vi "GUI_Single Button Pump.vi"() -> ()   [LabVIEW 2011] (continued)
        n648 = call "Generate User Event.vi"("Add(t)/Remove(f) Event"=w1664, "error in (no error)"=w1676, "User Event in"=w1677, "Status Array In"=w1679, "Error Codes"=w1678) -> ("error out"=w1675:errorcluster)  [unwired: 5 in, 1 out]
        n649 = case shown="\"HPBD\"" w1673 {
          tunnel: [w1683 "M123 Roughing Valve is NOT open.\nPlease perform corrective action\n and click on continue.\nClick Exit to abort GPM" ("message") "HPBD Roughing Valve is NOT open.\nPlease perform corrective action\n and click on continue.\nClick Exit to abort GPM" ("message") "OAP Roughing Valve is NOT open.\nPlease perform corrective action\n and click on continue.\nClick Exit to abort GPM" ("message") w1690 "BTL Roughing Valve is NOT open.\nPlease perform corrective action\n and click on continue.\nClick Exit to abort GPM" ("message") "TARGET Roughing Valve is NOT open.\nPlease perform corrective action\n and click on continue.\nClick Exit to abort GPM" ("message") "BTL2 Roughing Valve is NOT open.\nPlease perform corrective action\n and click on continue.\nClick Exit to abort GPM" ("message") "HPD Roughing Valve is NOT open.\nPlease perform corrective action\n and click on continue.\nClick Exit to abort GPM" ("message")] -> w1668
          tunnel: [w1683 "Main: Check Roughing Valve Status>>M123" "Main: Check Roughing Valve Status>>HPBD" "Main: Check Roughing Valve Status>>OAP" w1690 "Main: Check Roughing Valve Status>>BTL" "Main: Check Roughing Valve Status>>TARGET" "Main: Check Roughing Valve Status>>BTL2" "Main: Check Roughing Valve Status>>HPD"] -> w1662
          frame "False", Default {
            w1683 = ""
          }
          frame "M123" {
          }
          frame "HPBD" {
          }
          frame "OAP" {
          }
          frame "COMP" {
            w1690 = ""
          }
          frame "BTL" {
          }
          frame "TARGET" {
          }
          frame "BTL2" {
          }
          frame "HPD" {
          }
        }
        n650 = call "MID-VAC Timer.vi"("Action"=timerAction_typdef."Timer Running") -> ("TO"=w1671:bool)  [unwired: 10 in]
        n651 = And(x=w1664, y=w1671) -> (x .and. y?=w1670:bool)
        n652 = call "Generate TO event.vi"("Boolean"=w1670, "message"=w1668, "User Event in"=w1669) -> ()  [unwired: 9 in]
        n653 = Unbundle By Name(w1667) -> ("VI Refnum"=w1666:refnum<vi>)
        n654 = control-ref of="User Input Panel"() -> (w1665:refnum<vi>)
        n655 = call "Gen Next State based on user input.vi"("Next State IN"="", "Generate Event?"=w1664, "Idle State"=w1662, "Continue To Wait State"=w1662, "VI Refnum"=w1666, "SubPanel in"=w1665) -> ("Next State Out"=w1661:string)  [unwired: 5 in]
        n656 = call <vilib>:"Add State(s) to Queue__jki_lib_state_machine.vi"("State(s) in Front (\"\")"=w1661, "State(s) in (\"\")"=w1682) -> ("States Out"=w1681:string)  [unwired: 13 in]
      }
      frame "---------- Main: Roughing Pumps----------" {
      }
      frame "Main: Start Roughing Pumps" {
        # "Open Roughing Pumps on both systems"
        n657 = Unbundle By Name(w1708) -> ("Debug Mode?"=w1707:bool)
        n658 = case shown="False" w1707 {
          tunnel: w1715 -> [w1722 w1728]
          tunnel: [w1719 w1728] -> w1714
          tunnel: w1708 -> [w1718 _]
          frame False {
            w1727 = T33[] [enum."LB Start Roughing Pump ", enum."EC Start Roughing Pump"] items=["No Action", "Set GPM Mode LB", "EXIT GPM Mode LB", "Set GPM Mode EC", "EXIT GPM Mode EC", "Set GVM mode LB", "Set GVM Mode EC", "Open LB Backing Valve", "Open EC Backing Valve", "Open EC Roughing Valve", "Open LB Roughing Valve", "Open M123 Roughing Valve", "Close M123 Roughing Valve", "Open Compressor Roughing Valve", "Close Compressor Roughing Valve", "Open BeamDump Roughing Valve", "Close BeamDump Roughing Valve", "Open OAP Roughing Valve", "Close OAP Roughing Valve", "Open BTL Roughing Valve", "Close BTL Roughing Valve", "Open Target Roughing Valve", "Close Target Roughing Valve", "Open BTL2 Roughing Valve", "Close BTL2 Roughing Valve", "Open HPD Roughing Valve", "Close HPD Roughing Valve", "LB Start Roughing Pump ", "EC Start Roughing Pump", "Open COMP Turbo Backing Valve", "Open M123 Turbo Backing Valve", "Open OAP Turbo Backing Valve", "Open HPBD Turbo Backing Valve", "Open BLT Turbo Backing Valve", "Open TARGET1 Turbo Backing Valve", "Open TARGET2 Turbo Backing Valve", "Open BLT2 Turbo Backing Valve", "Open HPD Turbo Backing Valve", "LB Start Turbo Backing Pump", "EC Start Turbo Backing Pump", "Start COMP Turbo Pump", "Start M123 Turbo Pump", "Start OAP Turbo Pump", "Start BTL Turbo Pump", "Start TARGET1 Turbo Pump", "Start TARGET2 Turbo Pump", "Start BTL2 Turbo Pump", "Start HPD Turbo Pump", "Open COMP Turbo Gate Valve", "Open M123 Turbo Gate Valve", "Open OAP Turbo Gate Valve", "Open BTL Turbo Gate Valve", "Open TARGET1 Turbo Gate Valve", "Open TARGET2 Turbo Gate Valve", "Open BTL2 Turbo Gate Valve", "Open HPD Turbo Gate Valve"]
            n659 = Unbundle By Name(w1718) -> ("TCPConnection.Command TCP Connection EC"=w1723:refnum<k5>)
            n660 = Unbundle By Name(w1718) -> ("TCPConnection.Command TCP Connection LB"=w1725:refnum<k5>)
            n661 = call "Build Command.vi"("Command Array in"=w1727, "input cluster"=w1718) -> ("output EC Command cluster"=w1724:T34, "output LB Command cluster"=w1726:T34)  [unwired: 8 in]
            n662 = call "Send Command LB.vi"("error in (no error)"=w1722, "output LB Command cluster"=w1726, "TCP Network Connection in"=w1725) -> ("error out"=w1720:errorcluster)  [unwired: 8 in]
            n663 = call "Send Command EC.vi"("error in (no error)"=w1722, "output EC Command cluster"=w1724, "TCP Network Connection in"=w1723) -> ("error out"=w1721:errorcluster)  [unwired: 8 in]
            n664 = Merge Errors(w1720, w1721) -> (w1719:errorcluster)
          }
          frame True {
          }
        }
        n665 = call "Reset Command Clusters.vi"("error in (no error)"=w1714, "input cluster"=w1708) -> ("error out"=w1713:errorcluster, "output cluster"=w1712:T20)  [unwired: 8 in]
        n666 = call "MID-VAC Timer.vi"("TO sec (Start timer)"=300.0, "Action"=timerAction_typdef."Start Timer") -> ()  [unwired: 9 in, 1 out]
        n667 = call <vilib>:"Add State(s) to Queue__jki_lib_state_machine.vi"("State(s) in Front (\"\")"="Main: Check Roughing Pump Status", "State(s) in (\"\")"=w1717) -> ("States Out"=w1716:string)  [unwired: 13 in]
      }
      frame "Main: Check Roughing Pump Status" {
        w1733 = "Main: Check Roughing Pump Status"
        w1744 = Error_codes."011-Roughing Pump Status" ("Error Codes")
        w1747 = T32[] [enum."Is the EC Roughing Pump ON?", enum."Is the LB Roughing Pump ON?", enum."Does the EC Roughing Pump have a fault?", enum."Does the LB Roughing Pump have a fault?"] items=["No Action", "Is EC GPM Mode ON?", "Is EC GPM Mode Off?", "Is EC GVM Mode ON?", "Is EC GVM Off?", "Is  EC GPM or GVM Mode ON?", "Is LB GPM Mode ON?", "Is LB GPM Mode Off?", "Is LB GVM Mode ON?", "Is LB GVM Mode Off?", "Is  LB GPM or GVM Mode ON?", "Is M123 Turbo Gate Valve Opened? ", "Is M123 Turbo Gate Valve Closed?", "Is OAP Turbo Gate Valve Opened?", "Is OAP Turbo Gate Valve Closed?", "Is BTLTurbo Gate Valve Opened?", "Is BTL Turbo Gate Valve Closed?", "Is TARGET Turbo Gate Valve 1Opened?", "Is TARGET1 Turbo Gate Valve Closed?", "Is TARGET Turbo Gate Valve 2 Opened?", "Is TAREGT2 Turbo Gate Valve Closed?", "Is BTL2 Turbo Gate Valve Opened?", "Is BTL2 Turbo Gate Valve Closed?", "Is HPD Turbo Gate Valve Opened?", "Is HPD Turbo Gate Valve Closed?", "Is COMP to M123 gate Valve Opened?", "Is COMP to M123 Valve Closed?", "Is HPBD Gate Valve Opened?", "Is HPBD Gate Valve Closed?", "Is M123 to OAP gate valve opened?", "Is M123 to OAP gate valve closed?", "Is OAP to BLT gate valve opened?", "Is OAP to BTL Gate Valve Closed?", "Is BLT to TARGET gate valve opened?", "Is BTL to TARGET Gate Valve Closed?", "Is TARGET to BLT2 gate valve opened?", "Is TARGET to BTL2 Gate Valve Closed?", "Is BLT2 to HPD gate valve opened?", "Is BTL2 to HPD Gate Valve Closed?", "Is COMP at Atmospheric Pressure?", "Is M123 at Atmospheric Pressure?", "Is BeamDump at Atmospheric Pressure?", "Is OAP at Atmospheric Pressure?", "Is BLT at Atmospheric Pressure", "Is TARGET at Atmospheric Pressure?", "Is BLT2 at Atmospheric Pressure?", "Is HPD at Atmospheric Pressure?", "Is the EC Roughing Pump ON?", "Is the EC Roughing Pump OFF?", "Does the EC Roughing Pump have a fault?", "Is the LB Roughing Pump ON?", "Is the LB Roughing Pump Off?", "Does the LB Roughing Pump have a fault?", "Is the EC Backing Pump ON?", "Is the EC Backing Pump OFF?", "Is the LB Backing Pump ON?", "Is the LB Backing Pump OFF?", "Does the EC Backing Pump have a fault?", "Does the LB Backing Pump have a fault?", "Is the EC Backing Pipe at Atmospheric Pressure", "Is the LB Backing Pipe at Atmospheric Pressure", "Is the EC Backing Manifold at Atmospheric Pressure", "s the LB Backing Manifold at Atmospheric Pressure?", "Is the EC Roughing Pipe at Atmospheric Pressure", "Is the LB Roughing Pipe at Atmospheric Pressure?", "Is the EC Roughing Manifold at Atmospheric Pressure", "Is the LB Roughing Manifold at Atmospheric Pressure", "Is LB Backing Manifold Valve Opened?", "Is EC Backing Manifold Valve Opened?", "Is LB Roughing Manifold Valve Opened?", "Is EC Roughing Manifold Valve Opened?", "Is COMP Roughing Valve Opened?", "Is M123 Roughing Valve Opened?", "Is M123 Roughing Valve Closed?", "Is OAP Roughing Valve Opened?", "Is OAP Roughing Valve Closed?", "Is HPBD Roughing Valve Opened?", "Is HPBD Roughing Valve Closed?", "Is BTL Roughing Valve Opened?", "Is BTL Roughing Valve Closed?", "Is TARGET Roughing Valve Opened?", "Is TARGET Roughing Valve Closed?", "Is BTL2 Roughing Valve Opened?", "Is BTL2 Roughing Valve Closed?", "Is HPD Roughing Valve Opened?", "Is HPD Roughing Valve Closed?", "Is COMP Turbo Backing Valve Opened?", "Is M123 Turbo Backing Valve Opened", "Is HPBD Turbo Backing Valve Opened?", "Is OAP Turbo Backing Valve Opened?", "Is BTL Turbo Backing Valve Opened?", "Is TARGET1 Turbo Backing Valve Opened?", "Is TARGET2 Turbo Backing Valve Opened?", "Is BTL2 Turbo Backing Valve Opened?", "Is HPD Turbo Backing Valve Opened?", "Is M123 Backing at MID-VAC?", "Is OAP Backing at MID-VAC?", "Is TARGET1 Backing at MID-VAC?", "Is TARGET2 Backing at MID-VAC?", "Is BTL Backing at MID-VAC?", "Is BTL2 Backing at MID-VAC?", "Is HPD Backing at MID-VAC?", "Is M123 Turbo in Normal Operation", "Is COMP Turbo in Normal Operation", "Is OAP Turbo in Normal Operation", "Is BTL Turbo in Normal Operation", "Is TARGET1 Turbo in Normal Operation", "Is TARGET2 Turbo in Normal Operation", "Is BTL2 Turbo in Normal Operation", "Is HPD Turbo in Normal Operation", "Is M123 at MID-VAC?", "Is OAP at MID-VAC?", "Is COMP at MID-VAC?", "Is BTL at MID-VAC?", "Is TARGET at MID-VAC?", "Is BTL2 at MID-VAC?", "Is HPD at MID-VAC?"]
        # "If EC ON the no event\nIf LB ON then NO event\nIf EC No fauult then No event\nIf LB No fault then NO event"
        # "Event TAG"
        n668 = call "GetAction.vi"("Check Condition"=w1744, "Query Array"=w1747, "input cluster"=w1732, "error in (no error)"=w1746) -> ("Status Array Out"=w1745:string[], "Generate Event?"=w1731:bool, "error out"=w1742:errorcluster)  [unwired: 6 in, 3 out]
        n669 = call "Generate User Event.vi"("Add(t)/Remove(f) Event"=w1731, "error in (no error)"=w1742, "User Event in"=w1743, "Status Array In"=w1745, "Error Codes"=w1744) -> ("error out"=w1741:errorcluster)  [unwired: 5 in, 1 out]
        n670 = call "MID-VAC Timer.vi"("Action"=timerAction_typdef."Timer Running") -> ("TO"=w1739:bool)  [unwired: 10 in]
        n671 = And(x=w1731, y=w1739) -> (x .and. y?=w1738:bool)
        n672 = Unbundle By Name(w1732) -> ("VI Refnum"=w1736:refnum<vi>)
        n673 = control-ref of="User Input Panel"() -> (w1735:refnum<vi>)
        n674 = call "Generate TO event.vi"("Boolean"=w1738, "message"="Roughing Pump is NOT On or has a fault.\nPlease perform corrective action\n and click on continue.\nClick Exit to abort GPM", "User Event in"=w1737) -> ()  [unwired: 9 in]
        n675 = call "Gen Next State based on user input.vi"("Next State IN"="Main: Open Backing Manifold Valves", "Generate Event?"=w1731, "Idle State"=w1733, "Continue To Wait State"=w1733, "VI Refnum"=w1736, "SubPanel in"=w1735) -> ("Next State Out"=w1729:string)  [unwired: 5 in]
        n676 = call <vilib>:"Add State(s) to Queue__jki_lib_state_machine.vi"("State(s) in Front (\"\")"=w1729, "State(s) in (\"\")"=w1749) -> ("States Out"=w1748:string)  [unwired: 13 in]
      }
      frame "---------- Main: Backing Manifold ----------" {
      }
      frame "Main: Check Backing Pump Status" {
        w1759 = "Main: Check Backing Pump Status"
        w1768 = Error_codes."007-Backing Pump Status" ("Error Codes")
        w1771 = T32[] [enum."Is the EC Backing Pump OFF?", enum."Is the LB Backing Pump OFF?", enum."Does the EC Backing Pump have a fault?", enum."Does the LB Backing Pump have a fault?"] items=["No Action", "Is EC GPM Mode ON?", "Is EC GPM Mode Off?", "Is EC GVM Mode ON?", "Is EC GVM Off?", "Is  EC GPM or GVM Mode ON?", "Is LB GPM Mode ON?", "Is LB GPM Mode Off?", "Is LB GVM Mode ON?", "Is LB GVM Mode Off?", "Is  LB GPM or GVM Mode ON?", "Is M123 Turbo Gate Valve Opened? ", "Is M123 Turbo Gate Valve Closed?", "Is OAP Turbo Gate Valve Opened?", "Is OAP Turbo Gate Valve Closed?", "Is BTLTurbo Gate Valve Opened?", "Is BTL Turbo Gate Valve Closed?", "Is TARGET Turbo Gate Valve 1Opened?", "Is TARGET1 Turbo Gate Valve Closed?", "Is TARGET Turbo Gate Valve 2 Opened?", "Is TAREGT2 Turbo Gate Valve Closed?", "Is BTL2 Turbo Gate Valve Opened?", "Is BTL2 Turbo Gate Valve Closed?", "Is HPD Turbo Gate Valve Opened?", "Is HPD Turbo Gate Valve Closed?", "Is COMP to M123 gate Valve Opened?", "Is COMP to M123 Valve Closed?", "Is HPBD Gate Valve Opened?", "Is HPBD Gate Valve Closed?", "Is M123 to OAP gate valve opened?", "Is M123 to OAP gate valve closed?", "Is OAP to BLT gate valve opened?", "Is OAP to BTL Gate Valve Closed?", "Is BLT to TARGET gate valve opened?", "Is BTL to TARGET Gate Valve Closed?", "Is TARGET to BLT2 gate valve opened?", "Is TARGET to BTL2 Gate Valve Closed?", "Is BLT2 to HPD gate valve opened?", "Is BTL2 to HPD Gate Valve Closed?", "Is COMP at Atmospheric Pressure?", "Is M123 at Atmospheric Pressure?", "Is BeamDump at Atmospheric Pressure?", "Is OAP at Atmospheric Pressure?", "Is BLT at Atmospheric Pressure", "Is TARGET at Atmospheric Pressure?", "Is BLT2 at Atmospheric Pressure?", "Is HPD at Atmospheric Pressure?", "Is the EC Roughing Pump ON?", "Is the EC Roughing Pump OFF?", "Does the EC Roughing Pump have a fault?", "Is the LB Roughing Pump ON?", "Is the LB Roughing Pump Off?", "Does the LB Roughing Pump have a fault?", "Is the EC Backing Pump ON?", "Is the EC Backing Pump OFF?", "Is the LB Backing Pump ON?", "Is the LB Backing Pump OFF?", "Does the EC Backing Pump have a fault?", "Does the LB Backing Pump have a fault?", "Is the EC Backing Pipe at Atmospheric Pressure", "Is the LB Backing Pipe at Atmospheric Pressure", "Is the EC Backing Manifold at Atmospheric Pressure", "s the LB Backing Manifold at Atmospheric Pressure?", "Is the EC Roughing Pipe at Atmospheric Pressure", "Is the LB Roughing Pipe at Atmospheric Pressure?", "Is the EC Roughing Manifold at Atmospheric Pressure", "Is the LB Roughing Manifold at Atmospheric Pressure", "Is LB Backing Manifold Valve Opened?", "Is EC Backing Manifold Valve Opened?", "Is LB Roughing Manifold Valve Opened?", "Is EC Roughing Manifold Valve Opened?", "Is COMP Roughing Valve Opened?", "Is M123 Roughing Valve Opened?", "Is M123 Roughing Valve Closed?", "Is OAP Roughing Valve Opened?", "Is OAP Roughing Valve Closed?", "Is HPBD Roughing Valve Opened?", "Is HPBD Roughing Valve Closed?", "Is BTL Roughing Valve Opened?", "Is BTL Roughing Valve Closed?", "Is TARGET Roughing Valve Opened?", "Is TARGET Roughing Valve Closed?", "Is BTL2 Roughing Valve Opened?", "Is BTL2 Roughing Valve Closed?", "Is HPD Roughing Valve Opened?", "Is HPD Roughing Valve Closed?", "Is COMP Turbo Backing Valve Opened?", "Is M123 Turbo Backing Valve Opened", "Is HPBD Turbo Backing Valve Opened?", "Is OAP Turbo Backing Valve Opened?", "Is BTL Turbo Backing Valve Opened?", "Is TARGET1 Turbo Backing Valve Opened?", "Is TARGET2 Turbo Backing Valve Opened?", "Is BTL2 Turbo Backing Valve Opened?", "Is HPD Turbo Backing Valve Opened?", "Is M123 Backing at MID-VAC?", "Is OAP Backing at MID-VAC?", "Is TARGET1 Backing at MID-VAC?", "Is TARGET2 Backing at MID-VAC?", "Is BTL Backing at MID-VAC?", "Is BTL2 Backing at MID-VAC?", "Is HPD Backing at MID-VAC?", "Is M123 Turbo in Normal Operation", "Is COMP Turbo in Normal Operation", "Is OAP Turbo in Normal Operation", "Is BTL Turbo in Normal Operation", "Is TARGET1 Turbo in Normal Operation", "Is TARGET2 Turbo in Normal Operation", "Is BTL2 Turbo in Normal Operation", "Is HPD Turbo in Normal Operation", "Is M123 at MID-VAC?", "Is OAP at MID-VAC?", "Is COMP at MID-VAC?", "Is BTL at MID-VAC?", "Is TARGET at MID-VAC?", "Is BTL2 at MID-VAC?", "Is HPD at MID-VAC?"]
        # "Event TAG"
        n677 = call "GetAction.vi"("Check Condition"=w1768, "Query Array"=w1771, "input cluster"=w1754, "error in (no error)"=w1770) -> ("Status Array Out"=w1769:string[], "Generate Event?"=w1757:bool, "error out"=w1766:errorcluster)  [unwired: 6 in, 3 out]
        n678 = call "Generate User Event.vi"("Add(t)/Remove(f) Event"=w1757, "error in (no error)"=w1766, "User Event in"=w1767, "Status Array In"=w1769, "Error Codes"=w1768) -> ("error out"=w1765:errorcluster)  [unwired: 5 in, 1 out]
        n679 = call "MID-VAC Timer.vi"("Action"=timerAction_typdef."Timer Running") -> ("TO"=w1763:bool)  [unwired: 10 in]
        n680 = And(x=w1757, y=w1763) -> (x .and. y?=w1762:bool)
        n681 = Unbundle By Name(w1754) -> ("VI Refnum"=w1761:refnum<vi>)
        n682 = control-ref of="User Input Panel"() -> (w1760:refnum<vi>)
        n683 = call "Generate TO event.vi"("Boolean"=w1762, "message"="Backing Pump is On or has a fault.\nClick Continue to Wait for 30 Seconds.\nClick Exit to abort GPM", "User Event in"=w1756) -> ()  [unwired: 9 in]
        n684 = call "Gen Next State based on user input.vi"("Next State IN"="Main: Check Backing Manifold Pressure", "Generate Event?"=w1757, "Idle State"=w1759, "Continue To Wait State"=w1759, "VI Refnum"=w1761, "SubPanel in"=w1760) -> ("Next State Out"=w1755:string)  [unwired: 5 in]
        n685 = call <vilib>:"Add State(s) to Queue__jki_lib_state_machine.vi"("State(s) in (\"\")"=w1773, "State(s) at Back (\"\")"=w1755) -> ("States Out"=w1772:string)  [unwired: 13 in]
      }
      frame "Main: Check Backing Manifold Pressure" {
        w1780 = "Main: Check Backing Manifold Pressure"
        w1789 = Error_codes."007-Backing Pump Status" ("Error Codes")
        w1792 = T32[] [enum."Is the EC Backing Pipe at Atmospheric Pressure", enum."Is the EC Backing Manifold at Atmospheric Pressure", enum."Is the LB Backing Pipe at Atmospheric Pressure", enum."s the LB Backing Manifold at Atmospheric Pressure?"] items=["No Action", "Is EC GPM Mode ON?", "Is EC GPM Mode Off?", "Is EC GVM Mode ON?", "Is EC GVM Off?", "Is  EC GPM or GVM Mode ON?", "Is LB GPM Mode ON?", "Is LB GPM Mode Off?", "Is LB GVM Mode ON?", "Is LB GVM Mode Off?", "Is  LB GPM or GVM Mode ON?", "Is M123 Turbo Gate Valve Opened? ", "Is M123 Turbo Gate Valve Closed?", "Is OAP Turbo Gate Valve Opened?", "Is OAP Turbo Gate Valve Closed?", "Is BTLTurbo Gate Valve Opened?", "Is BTL Turbo Gate Valve Closed?", "Is TARGET Turbo Gate Valve 1Opened?", "Is TARGET1 Turbo Gate Valve Closed?", "Is TARGET Turbo Gate Valve 2 Opened?", "Is TAREGT2 Turbo Gate Valve Closed?", "Is BTL2 Turbo Gate Valve Opened?", "Is BTL2 Turbo Gate Valve Closed?", "Is HPD Turbo Gate Valve Opened?", "Is HPD Turbo Gate Valve Closed?", "Is COMP to M123 gate Valve Opened?", "Is COMP to M123 Valve Closed?", "Is HPBD Gate Valve Opened?", "Is HPBD Gate Valve Closed?", "Is M123 to OAP gate valve opened?", "Is M123 to OAP gate valve closed?", "Is OAP to BLT gate valve opened?", "Is OAP to BTL Gate Valve Closed?", "Is BLT to TARGET gate valve opened?", "Is BTL to TARGET Gate Valve Closed?", "Is TARGET to BLT2 gate valve opened?", "Is TARGET to BTL2 Gate Valve Closed?", "Is BLT2 to HPD gate valve opened?", "Is BTL2 to HPD Gate Valve Closed?", "Is COMP at Atmospheric Pressure?", "Is M123 at Atmospheric Pressure?", "Is BeamDump at Atmospheric Pressure?", "Is OAP at Atmospheric Pressure?", "Is BLT at Atmospheric Pressure", "Is TARGET at Atmospheric Pressure?", "Is BLT2 at Atmospheric Pressure?", "Is HPD at Atmospheric Pressure?", "Is the EC Roughing Pump ON?", "Is the EC Roughing Pump OFF?", "Does the EC Roughing Pump have a fault?", "Is the LB Roughing Pump ON?", "Is the LB Roughing Pump Off?", "Does the LB Roughing Pump have a fault?", "Is the EC Backing Pump ON?", "Is the EC Backing Pump OFF?", "Is the LB Backing Pump ON?", "Is the LB Backing Pump OFF?", "Does the EC Backing Pump have a fault?", "Does the LB Backing Pump have a fault?", "Is the EC Backing Pipe at Atmospheric Pressure", "Is the LB Backing Pipe at Atmospheric Pressure", "Is the EC Backing Manifold at Atmospheric Pressure", "s the LB Backing Manifold at Atmospheric Pressure?", "Is the EC Roughing Pipe at Atmospheric Pressure", "Is the LB Roughing Pipe at Atmospheric Pressure?", "Is the EC Roughing Manifold at Atmospheric Pressure", "Is the LB Roughing Manifold at Atmospheric Pressure", "Is LB Backing Manifold Valve Opened?", "Is EC Backing Manifold Valve Opened?", "Is LB Roughing Manifold Valve Opened?", "Is EC Roughing Manifold Valve Opened?", "Is COMP Roughing Valve Opened?", "Is M123 Roughing Valve Opened?", "Is M123 Roughing Valve Closed?", "Is OAP Roughing Valve Opened?", "Is OAP Roughing Valve Closed?", "Is HPBD Roughing Valve Opened?", "Is HPBD Roughing Valve Closed?", "Is BTL Roughing Valve Opened?", "Is BTL Roughing Valve Closed?", "Is TARGET Roughing Valve Opened?", "Is TARGET Roughing Valve Closed?", "Is BTL2 Roughing Valve Opened?", "Is BTL2 Roughing Valve Closed?", "Is HPD Roughing Valve Opened?", "Is HPD Roughing Valve Closed?", "Is COMP Turbo Backing Valve Opened?", "Is M123 Turbo Backing Valve Opened", "Is HPBD Turbo Backing Valve Opened?", "Is OAP Turbo Backing Valve Opened?", "Is BTL Turbo Backing Valve Opened?", "Is TARGET1 Turbo Backing Valve Opened?", "Is TARGET2 Turbo Backing Valve Opened?", "Is BTL2 Turbo Backing Valve Opened?", "Is HPD Turbo Backing Valve Opened?", "Is M123 Backing at MID-VAC?", "Is OAP Backing at MID-VAC?", "Is TARGET1 Backing at MID-VAC?", "Is TARGET2 Backing at MID-VAC?", "Is BTL Backing at MID-VAC?", "Is BTL2 Backing at MID-VAC?", "Is HPD Backing at MID-VAC?", "Is M123 Turbo in Normal Operation", "Is COMP Turbo in Normal Operation", "Is OAP Turbo in Normal Operation", "Is BTL Turbo in Normal Operation", "Is TARGET1 Turbo in Normal Operation", "Is TARGET2 Turbo in Normal Operation", "Is BTL2 Turbo in Normal Operation", "Is HPD Turbo in Normal Operation", "Is M123 at MID-VAC?", "Is OAP at MID-VAC?", "Is COMP at MID-VAC?", "Is BTL at MID-VAC?", "Is TARGET at MID-VAC?", "Is BTL2 at MID-VAC?", "Is HPD at MID-VAC?"]
        # "Event TAG"
        n686 = call "GetAction.vi"("Check Condition"=w1789, "Query Array"=w1792, "input cluster"=w1775, "error in (no error)"=w1791) -> ("Status Array Out"=w1790:string[], "Generate Event?"=w1777:bool, "error out"=w1787:errorcluster)  [unwired: 6 in, 3 out]
        n687 = call "Generate User Event.vi"("Add(t)/Remove(f) Event"=w1777, "error in (no error)"=w1787, "User Event in"=w1788, "Status Array In"=w1790, "Error Codes"=w1789) -> ("error out"=w1786:errorcluster)  [unwired: 5 in, 1 out]
        n688 = call "MID-VAC Timer.vi"("Action"=timerAction_typdef."Timer Running") -> ("TO"=w1784:bool)  [unwired: 10 in]
        n689 = And(x=w1777, y=w1784) -> (x .and. y?=w1783:bool)
        n690 = Unbundle By Name(w1775) -> ("VI Refnum"=w1782:refnum<vi>)
        n691 = control-ref of="User Input Panel"() -> (w1781:refnum<vi>)
        n692 = call "Generate TO event.vi"("Boolean"=w1783, "message"="Backing Pipe and Manifold are not Vented\nPlease perform corrective action\n and click on continue.\nClick Exit to abort GPM", "User Event in"=w1778) -> ()  [unwired: 9 in]
        n693 = call "Gen Next State based on user input.vi"("Next State IN"="Main: Open Backing Manifold Valves", "Generate Event?"=w1777, "Idle State"=w1780, "Continue To Wait State"=w1780, "VI Refnum"=w1782, "SubPanel in"=w1781) -> ("Next State Out"=w1776:string)  [unwired: 5 in]
        n694 = call <vilib>:"Add State(s) to Queue__jki_lib_state_machine.vi"("State(s) in (\"\")"=w1794, "State(s) at Back (\"\")"=w1776) -> ("States Out"=w1793:string)  [unwired: 13 in]
      }
      frame "Main: Open Backing Manifold Valves" {
        # "Open Backing Valves on both systems"
        n695 = Unbundle By Name(w1796) -> ("Debug Mode?"=w1795:bool)
        n696 = case shown="False" w1795 {
          tunnel: w1801 -> [w1808 w1814]
          tunnel: [w1805 w1814] -> w1799
          tunnel: w1796 -> [w1804 _]
          frame False {
            w1813 = T33[] [enum."Open LB Backing Valve", enum."Open EC Backing Valve"] items=["No Action", "Set GPM Mode LB", "EXIT GPM Mode LB", "Set GPM Mode EC", "EXIT GPM Mode EC", "Set GVM mode LB", "Set GVM Mode EC", "Open LB Backing Valve", "Open EC Backing Valve", "Open EC Roughing Valve", "Open LB Roughing Valve", "Open M123 Roughing Valve", "Close M123 Roughing Valve", "Open Compressor Roughing Valve", "Close Compressor Roughing Valve", "Open BeamDump Roughing Valve", "Close BeamDump Roughing Valve", "Open OAP Roughing Valve", "Close OAP Roughing Valve", "Open BTL Roughing Valve", "Close BTL Roughing Valve", "Open Target Roughing Valve", "Close Target Roughing Valve", "Open BTL2 Roughing Valve", "Close BTL2 Roughing Valve", "Open HPD Roughing Valve", "Close HPD Roughing Valve", "LB Start Roughing Pump ", "EC Start Roughing Pump", "Open COMP Turbo Backing Valve", "Open M123 Turbo Backing Valve", "Open OAP Turbo Backing Valve", "Open HPBD Turbo Backing Valve", "Open BLT Turbo Backing Valve", "Open TARGET1 Turbo Backing Valve", "Open TARGET2 Turbo Backing Valve", "Open BLT2 Turbo Backing Valve", "Open HPD Turbo Backing Valve", "LB Start Turbo Backing Pump", "EC Start Turbo Backing Pump", "Start COMP Turbo Pump", "Start M123 Turbo Pump", "Start OAP Turbo Pump", "Start BTL Turbo Pump", "Start TARGET1 Turbo Pump", "Start TARGET2 Turbo Pump", "Start BTL2 Turbo Pump", "Start HPD Turbo Pump", "Open COMP Turbo Gate Valve", "Open M123 Turbo Gate Valve", "Open OAP Turbo Gate Valve", "Open BTL Turbo Gate Valve", "Open TARGET1 Turbo Gate Valve", "Open TARGET2 Turbo Gate Valve", "Open BTL2 Turbo Gate Valve", "Open HPD Turbo Gate Valve"]
            n697 = Unbundle By Name(w1804) -> ("TCPConnection.Command TCP Connection EC"=w1809:refnum<k5>)
            n698 = Unbundle By Name(w1804) -> ("TCPConnection.Command TCP Connection LB"=w1811:refnum<k5>)
            n699 = call "Build Command.vi"("Command Array in"=w1813, "input cluster"=w1804) -> ("output EC Command cluster"=w1810:T34, "output LB Command cluster"=w1812:T34)  [unwired: 8 in]
            n700 = call "Send Command LB.vi"("error in (no error)"=w1808, "output LB Command cluster"=w1812, "TCP Network Connection in"=w1811) -> ("error out"=w1806:errorcluster)  [unwired: 8 in]
            n701 = call "Send Command EC.vi"("error in (no error)"=w1808, "output EC Command cluster"=w1810, "TCP Network Connection in"=w1809) -> ("error out"=w1807:errorcluster)  [unwired: 8 in]
            n702 = Merge Errors(w1806, w1807) -> (w1805:errorcluster)
          }
          frame True {
          }
        }
        n703 = call "Reset Command Clusters.vi"("error in (no error)"=w1799, "input cluster"=w1796) -> ("error out"=w1798:errorcluster, "output cluster"=w1797:T20)  [unwired: 8 in]
        n704 = call <vilib>:"Add State(s) to Queue__jki_lib_state_machine.vi"("State(s) in Front (\"\")"="Main: Check Backing Manifold Valve Status", "State(s) in (\"\")"=w1803) -> ("States Out"=w1802:string)  [unwired: 13 in]
      }
      frame "Main: Check Backing Manifold Valve Status" {
        w1821 = "Main: Check Backing Manifold Valve Status"
        w1830 = Error_codes."008-Backing valve status" ("Error Codes")
        w1833 = T32[] [enum."Is LB Backing Manifold Valve Opened?", enum."Is EC Backing Manifold Valve Opened?"] items=["No Action", "Is EC GPM Mode ON?", "Is EC GPM Mode Off?", "Is EC GVM Mode ON?", "Is EC GVM Off?", "Is  EC GPM or GVM Mode ON?", "Is LB GPM Mode ON?", "Is LB GPM Mode Off?", "Is LB GVM Mode ON?", "Is LB GVM Mode Off?", "Is  LB GPM or GVM Mode ON?", "Is M123 Turbo Gate Valve Opened? ", "Is M123 Turbo Gate Valve Closed?", "Is OAP Turbo Gate Valve Opened?", "Is OAP Turbo Gate Valve Closed?", "Is BTLTurbo Gate Valve Opened?", "Is BTL Turbo Gate Valve Closed?", "Is TARGET Turbo Gate Valve 1Opened?", "Is TARGET1 Turbo Gate Valve Closed?", "Is TARGET Turbo Gate Valve 2 Opened?", "Is TAREGT2 Turbo Gate Valve Closed?", "Is BTL2 Turbo Gate Valve Opened?", "Is BTL2 Turbo Gate Valve Closed?", "Is HPD Turbo Gate Valve Opened?", "Is HPD Turbo Gate Valve Closed?", "Is COMP to M123 gate Valve Opened?", "Is COMP to M123 Valve Closed?", "Is HPBD Gate Valve Opened?", "Is HPBD Gate Valve Closed?", "Is M123 to OAP gate valve opened?", "Is M123 to OAP gate valve closed?", "Is OAP to BLT gate valve opened?", "Is OAP to BTL Gate Valve Closed?", "Is BLT to TARGET gate valve opened?", "Is BTL to TARGET Gate Valve Closed?", "Is TARGET to BLT2 gate valve opened?", "Is TARGET to BTL2 Gate Valve Closed?", "Is BLT2 to HPD gate valve opened?", "Is BTL2 to HPD Gate Valve Closed?", "Is COMP at Atmospheric Pressure?", "Is M123 at Atmospheric Pressure?", "Is BeamDump at Atmospheric Pressure?", "Is OAP at Atmospheric Pressure?", "Is BLT at Atmospheric Pressure", "Is TARGET at Atmospheric Pressure?", "Is BLT2 at Atmospheric Pressure?", "Is HPD at Atmospheric Pressure?", "Is the EC Roughing Pump ON?", "Is the EC Roughing Pump OFF?", "Does the EC Roughing Pump have a fault?", "Is the LB Roughing Pump ON?", "Is the LB Roughing Pump Off?", "Does the LB Roughing Pump have a fault?", "Is the EC Backing Pump ON?", "Is the EC Backing Pump OFF?", "Is the LB Backing Pump ON?", "Is the LB Backing Pump OFF?", "Does the EC Backing Pump have a fault?", "Does the LB Backing Pump have a fault?", "Is the EC Backing Pipe at Atmospheric Pressure", "Is the LB Backing Pipe at Atmospheric Pressure", "Is the EC Backing Manifold at Atmospheric Pressure", "s the LB Backing Manifold at Atmospheric Pressure?", "Is the EC Roughing Pipe at Atmospheric Pressure", "Is the LB Roughing Pipe at Atmospheric Pressure?", "Is the EC Roughing Manifold at Atmospheric Pressure", "Is the LB Roughing Manifold at Atmospheric Pressure", "Is LB Backing Manifold Valve Opened?", "Is EC Backing Manifold Valve Opened?", "Is LB Roughing Manifold Valve Opened?", "Is EC Roughing Manifold Valve Opened?", "Is COMP Roughing Valve Opened?", "Is M123 Roughing Valve Opened?", "Is M123 Roughing Valve Closed?", "Is OAP Roughing Valve Opened?", "Is OAP Roughing Valve Closed?", "Is HPBD Roughing Valve Opened?", "Is HPBD Roughing Valve Closed?", "Is BTL Roughing Valve Opened?", "Is BTL Roughing Valve Closed?", "Is TARGET Roughing Valve Opened?", "Is TARGET Roughing Valve Closed?", "Is BTL2 Roughing Valve Opened?", "Is BTL2 Roughing Valve Closed?", "Is HPD Roughing Valve Opened?", "Is HPD Roughing Valve Closed?", "Is COMP Turbo Backing Valve Opened?", "Is M123 Turbo Backing Valve Opened", "Is HPBD Turbo Backing Valve Opened?", "Is OAP Turbo Backing Valve Opened?", "Is BTL Turbo Backing Valve Opened?", "Is TARGET1 Turbo Backing Valve Opened?", "Is TARGET2 Turbo Backing Valve Opened?", "Is BTL2 Turbo Backing Valve Opened?", "Is HPD Turbo Backing Valve Opened?", "Is M123 Backing at MID-VAC?", "Is OAP Backing at MID-VAC?", "Is TARGET1 Backing at MID-VAC?", "Is TARGET2 Backing at MID-VAC?", "Is BTL Backing at MID-VAC?", "Is BTL2 Backing at MID-VAC?", "Is HPD Backing at MID-VAC?", "Is M123 Turbo in Normal Operation", "Is COMP Turbo in Normal Operation", "Is OAP Turbo in Normal Operation", "Is BTL Turbo in Normal Operation", "Is TARGET1 Turbo in Normal Operation", "Is TARGET2 Turbo in Normal Operation", "Is BTL2 Turbo in Normal Operation", "Is HPD Turbo in Normal Operation", "Is M123 at MID-VAC?", "Is OAP at MID-VAC?", "Is COMP at MID-VAC?", "Is BTL at MID-VAC?", "Is TARGET at MID-VAC?", "Is BTL2 at MID-VAC?", "Is HPD at MID-VAC?"]
        # "Event TAG"
        n705 = call "GetAction.vi"("Check Condition"=w1830, "Query Array"=w1833, "input cluster"=w1816, "error in (no error)"=w1832) -> ("Status Array Out"=w1831:string[], "Generate Event?"=w1818:bool, "error out"=w1828:errorcluster)  [unwired: 6 in, 3 out]
        n706 = call "Generate User Event.vi"("Add(t)/Remove(f) Event"=w1818, "error in (no error)"=w1828, "User Event in"=w1829, "Status Array In"=w1831, "Error Codes"=w1830) -> ("error out"=w1827:errorcluster)  [unwired: 5 in, 1 out]
        n707 = call "MID-VAC Timer.vi"("Action"=timerAction_typdef."Timer Running") -> ("TO"=w1825:bool)  [unwired: 10 in]
        n708 = And(x=w1818, y=w1825) -> (x .and. y?=w1824:bool)
        n709 = Unbundle By Name(w1816) -> ("VI Refnum"=w1823:refnum<vi>)
        n710 = control-ref of="User Input Panel"() -> (w1822:refnum<vi>)
        n711 = call "Generate TO event.vi"("Boolean"=w1824, "message"="Backing Manifold Valve is NOT open\nPlease perform corrective action\nClick on continue. to wait for 30 seconds more.\nClick Exit to abort GPM", "User Event in"=w1819) -> ()  [unwired: 9 in]
        n712 = call "Gen Next State based on user input.vi"("Next State IN"="Main: Open Turbo Backing Valves", "Generate Event?"=w1818, "Idle State"=w1821, "Continue To Wait State"=w1821, "VI Refnum"=w1823, "SubPanel in"=w1822) -> ("Next State Out"=w1817:string)  [unwired: 5 in]
        n713 = call <vilib>:"Add State(s) to Queue__jki_lib_state_machine.vi"("State(s) in (\"\")"=w1835, "State(s) at Back (\"\")"=w1817) -> ("States Out"=w1834:string)  [unwired: 13 in]
      }
      frame "---------- Main:Turbo Backing Valves ---------" {
      }
      frame "Main: Open Turbo Backing Valves" {
        # "Open Backing Valves on both systems"
        n714 = Unbundle By Name(w1842) -> ("Debug Mode?"=w1841:bool)
        n715 = case shown="False" w1841 {
          tunnel: w1847 -> [w1858 w1863]
          tunnel: [w1855 w1863] -> w1845
          tunnel: w1842 -> [w1851 _]
          frame False {
            n716 = Unbundle By Name(w1851) -> ("Chamber Selection"=w1854:T21, "Isolate HPBD"=w1850:bool)
            n717 = call "Selection ActionBuilder.vi"("Selection Action"=Selection_Action_typdef."Open Turbo Backing Valves", "Isolate HPBD"=w1850, "Chamber Selection"=w1854) -> ("Command Array Out"=w1852:T33[])  [unwired: 7 in, 1 out]
            n718 = Unbundle By Name(w1851) -> ("TCPConnection.Command TCP Connection EC"=w1859:refnum<k5>)
            n719 = Unbundle By Name(w1851) -> ("TCPConnection.Command TCP Connection LB"=w1861:refnum<k5>)
            n720 = call "Build Command.vi"("Command Array in"=w1852, "input cluster"=w1851) -> ("output EC Command cluster"=w1860:T34, "output LB Command cluster"=w1862:T34)  [unwired: 8 in]
            n721 = call "Send Command LB.vi"("error in (no error)"=w1858, "output LB Command cluster"=w1862, "TCP Network Connection in"=w1861) -> ("error out"=w1856:errorcluster)  [unwired: 8 in]
            n722 = call "Send Command EC.vi"("error in (no error)"=w1858, "output EC Command cluster"=w1860, "TCP Network Connection in"=w1859) -> ("error out"=w1857:errorcluster)  [unwired: 8 in]
            n723 = Merge Errors(w1856, w1857) -> (w1855:errorcluster)
          }
          frame True {
          }
        }
        n724 = call "Reset Command Clusters.vi"("error in (no error)"=w1845, "input cluster"=w1842) -> ("error out"=w1844:errorcluster, "output cluster"=w1843:T20)  [unwired: 8 in]
        n725 = call <vilib>:"Add State(s) to Queue__jki_lib_state_machine.vi"("State(s) in Front (\"\")"="Main: Check Turbo Backing Valve Status", "State(s) in (\"\")"=w1849) -> ("States Out"=w1848:string)  [unwired: 13 in]
        n726 = call "MID-VAC Timer.vi"("TO sec (Start timer)"=5.0, "Action"=timerAction_typdef."Start Timer") -> ()  [unwired: 9 in, 1 out]
      }
      frame "Main: Check Turbo Backing Valves Status" {
        w1868 = "Main: Check Turbo Backing Valves Status"
        w1882 = Error_codes."012-Turbo Backing Valve Status" ("Error Codes")
        # "Event TAG"
        n727 = Unbundle By Name(w1865) -> ("Chamber Selection"=w1874:T21, "Isolate HPBD"=w1872:bool)
        n728 = call "Selection ActionBuilder.vi"("Selection Action"=Selection_Action_typdef."Check Turbo Backing Valves", "Isolate HPBD"=w1872, "Chamber Selection"=w1874) -> ("Action Array Out"=w1864:T32[])  [unwired: 7 in, 1 out]
        n729 = call "GetAction.vi"("Check Condition"=w1882, "Query Array"=w1864, "input cluster"=w1865, "error in (no error)"=w1884) -> ("Status Array Out"=w1883:string[], "Generate Event?"=w1867:bool, "error out"=w1880:errorcluster)  [unwired: 6 in, 3 out]
        n730 = call "Generate User Event.vi"("Add(t)/Remove(f) Event"=w1867, "error in (no error)"=w1880, "User Event in"=w1881, "Status Array In"=w1883, "Error Codes"=w1882) -> ("error out"=w1879:errorcluster)  [unwired: 5 in, 1 out]
        n731 = call "MID-VAC Timer.vi"("Action"=timerAction_typdef."Timer Running") -> ("TO"=w1877:bool)  [unwired: 10 in]
        n732 = Unbundle By Name(w1865) -> ("VI Refnum"=w1870:refnum<vi>)
        n733 = control-ref of="User Input Panel"() -> (w1869:refnum<vi>)
        n734 = And(x=w1867, y=w1877) -> (x .and. y?=w1876:bool)
        n735 = call "Gen Next State based on user input.vi"("Next State IN"="Main: Start Turbo Backing Pump", "Generate Event?"=w1867, "Idle State"=w1868, "Continue To Wait State"=w1868, "VI Refnum"=w1870, "SubPanel in"=w1869) -> ()  [unwired: 5 in, 1 out]
        n736 = call "Generate TO event.vi"("Boolean"=w1876, "message"="Some Turbo Backing Valves are closed.\nPlease perform corrective action\n and click on continue.\nClick Exit to abort GPM", "User Event in"=w1871) -> ()  [unwired: 9 in]
        n737 = call <vilib>:"Add State(s) to Queue__jki_lib_state_machine.vi"("State(s) in (\"\")"=w1886) -> ("States Out"=w1885:string)  [unwired: 14 in]
      }
      frame "Main: Start Turbo Backing Pump" {
        # "Open Backing Valves on both systems"
        n738 = Unbundle By Name(w1888) -> ("Debug Mode?"=w1887:bool)
        n739 = case shown="False" w1887 {
          tunnel: w1893 -> [w1904 w1909]
          tunnel: [w1901 w1909] -> w1891
          tunnel: w1888 -> [w1897 _]
          frame False {
            w1899 = T33[] [enum."EC Start Turbo Backing Pump"] items=["No Action", "Set GPM Mode LB", "EXIT GPM Mode LB", "Set GPM Mode EC", "EXIT GPM Mode EC", "Set GVM mode LB", "Set GVM Mode EC", "Open LB Backing Valve", "Open EC Backing Valve", "Open EC Roughing Valve", "Open LB Roughing Valve", "Open M123 Roughing Valve", "Close M123 Roughing Valve", "Open Compressor Roughing Valve", "Close Compressor Roughing Valve", "Open BeamDump Roughing Valve", "Close BeamDump Roughing Valve", "Open OAP Roughing Valve", "Close OAP Roughing Valve", "Open BTL Roughing Valve", "Close BTL Roughing Valve", "Open Target Roughing Valve", "Close Target Roughing Valve", "Open BTL2 Roughing Valve", "Close BTL2 Roughing Valve", "Open HPD Roughing Valve", "Close HPD Roughing Valve", "LB Start Roughing Pump ", "EC Start Roughing Pump", "Open COMP Turbo Backing Valve", "Open M123 Turbo Backing Valve", "Open OAP Turbo Backing Valve", "Open HPBD Turbo Backing Valve", "Open BLT Turbo Backing Valve", "Open TARGET1 Turbo Backing Valve", "Open TARGET2 Turbo Backing Valve", "Open BLT2 Turbo Backing Valve", "Open HPD Turbo Backing Valve", "LB Start Turbo Backing Pump", "EC Start Turbo Backing Pump", "Start COMP Turbo Pump", "Start M123 Turbo Pump", "Start OAP Turbo Pump", "Start BTL Turbo Pump", "Start TARGET1 Turbo Pump", "Start TARGET2 Turbo Pump", "Start BTL2 Turbo Pump", "Start HPD Turbo Pump", "Open COMP Turbo Gate Valve", "Open M123 Turbo Gate Valve", "Open OAP Turbo Gate Valve", "Open BTL Turbo Gate Valve", "Open TARGET1 Turbo Gate Valve", "Open TARGET2 Turbo Gate Valve", "Open BTL2 Turbo Gate Valve", "Open HPD Turbo Gate Valve"]
            w1900 = T33[] [enum."LB Start Turbo Backing Pump"] items=["No Action", "Set GPM Mode LB", "EXIT GPM Mode LB", "Set GPM Mode EC", "EXIT GPM Mode EC", "Set GVM mode LB", "Set GVM Mode EC", "Open LB Backing Valve", "Open EC Backing Valve", "Open EC Roughing Valve", "Open LB Roughing Valve", "Open M123 Roughing Valve", "Close M123 Roughing Valve", "Open Compressor Roughing Valve", "Close Compressor Roughing Valve", "Open BeamDump Roughing Valve", "Close BeamDump Roughing Valve", "Open OAP Roughing Valve", "Close OAP Roughing Valve", "Open BTL Roughing Valve", "Close BTL Roughing Valve", "Open Target Roughing Valve", "Close Target Roughing Valve", "Open BTL2 Roughing Valve", "Close BTL2 Roughing Valve", "Open HPD Roughing Valve", "Close HPD Roughing Valve", "LB Start Roughing Pump ", "EC Start Roughing Pump", "Open COMP Turbo Backing Valve", "Open M123 Turbo Backing Valve", "Open OAP Turbo Backing Valve", "Open HPBD Turbo Backing Valve", "Open BLT Turbo Backing Valve", "Open TARGET1 Turbo Backing Valve", "Open TARGET2 Turbo Backing Valve", "Open BLT2 Turbo Backing Valve", "Open HPD Turbo Backing Valve", "LB Start Turbo Backing Pump", "EC Start Turbo Backing Pump", "Start COMP Turbo Pump", "Start M123 Turbo Pump", "Start OAP Turbo Pump", "Start BTL Turbo Pump", "Start TARGET1 Turbo Pump", "Start TARGET2 Turbo Pump", "Start BTL2 Turbo Pump", "Start HPD Turbo Pump", "Open COMP Turbo Gate Valve", "Open M123 Turbo Gate Valve", "Open OAP Turbo Gate Valve", "Open BTL Turbo Gate Valve", "Open TARGET1 Turbo Gate Valve", "Open TARGET2 Turbo Gate Valve", "Open BTL2 Turbo Gate Valve", "Open HPD Turbo Gate Valve"]
            n740 = Unbundle By Name(w1897) -> ("Chamber Selection"=w1896:T21)
            n741 = call "Selection ActionBuilder sections.vi"("EC Command Array"=w1899, "Chamber Selection"=w1896, "LB Command Array"=w1900) -> ("Command Array out"=w1898:T33[])  [unwired: 7 in, 1 out]
            n742 = Unbundle By Name(w1897) -> ("TCPConnection.Command TCP Connection EC"=w1905:refnum<k5>)
            n743 = Unbundle By Name(w1897) -> ("TCPConnection.Command TCP Connection LB"=w1907:refnum<k5>)
            n744 = call "Build Command.vi"("Command Array in"=w1898, "input cluster"=w1897) -> ("output EC Command cluster"=w1906:T34, "output LB Command cluster"=w1908:T34)  [unwired: 8 in]
            n745 = call "Send Command LB.vi"("error in (no error)"=w1904, "output LB Command cluster"=w1908, "TCP Network Connection in"=w1907) -> ("error out"=w1902:errorcluster)  [unwired: 8 in]
            n746 = call "Send Command EC.vi"("error in (no error)"=w1904, "output EC Command cluster"=w1906, "TCP Network Connection in"=w1905) -> ("error out"=w1903:errorcluster)  [unwired: 8 in]
            n747 = Merge Errors(w1902, w1903) -> (w1901:errorcluster)
          }
          frame True {
          }
        }
        n748 = call "Reset Command Clusters.vi"("error in (no error)"=w1891, "input cluster"=w1888) -> ("error out"=w1890:errorcluster, "output cluster"=w1889:T20)  [unwired: 8 in]
        n749 = call <vilib>:"Add State(s) to Queue__jki_lib_state_machine.vi"("State(s) in Front (\"\")"="Main: Wait for Backing Pump", "State(s) in (\"\")"=w1895) -> ("States Out"=w1894:string)  [unwired: 13 in]
      }
      frame "Main: Wait for Backing Pump" {
        w1911 = T32[] [enum."Is the LB Backing Pump ON?", enum."Does the LB Backing Pump have a fault?"] items=["No Action", "Is EC GPM Mode ON?", "Is EC GPM Mode Off?", "Is EC GVM Mode ON?", "Is EC GVM Off?", "Is  EC GPM or GVM Mode ON?", "Is LB GPM Mode ON?", "Is LB GPM Mode Off?", "Is LB GVM Mode ON?", "Is LB GVM Mode Off?", "Is  LB GPM or GVM Mode ON?", "Is M123 Turbo Gate Valve Opened? ", "Is M123 Turbo Gate Valve Closed?", "Is OAP Turbo Gate Valve Opened?", "Is OAP Turbo Gate Valve Closed?", "Is BTLTurbo Gate Valve Opened?", "Is BTL Turbo Gate Valve Closed?", "Is TARGET Turbo Gate Valve 1Opened?", "Is TARGET1 Turbo Gate Valve Closed?", "Is TARGET Turbo Gate Valve 2 Opened?", "Is TAREGT2 Turbo Gate Valve Closed?", "Is BTL2 Turbo Gate Valve Opened?", "Is BTL2 Turbo Gate Valve Closed?", "Is HPD Turbo Gate Valve Opened?", "Is HPD Turbo Gate Valve Closed?", "Is COMP to M123 gate Valve Opened?", "Is COMP to M123 Valve Closed?", "Is HPBD Gate Valve Opened?", "Is HPBD Gate Valve Closed?", "Is M123 to OAP gate valve opened?", "Is M123 to OAP gate valve closed?", "Is OAP to BLT gate valve opened?", "Is OAP to BTL Gate Valve Closed?", "Is BLT to TARGET gate valve opened?", "Is BTL to TARGET Gate Valve Closed?", "Is TARGET to BLT2 gate valve opened?", "Is TARGET to BTL2 Gate Valve Closed?", "Is BLT2 to HPD gate valve opened?", "Is BTL2 to HPD Gate Valve Closed?", "Is COMP at Atmospheric Pressure?", "Is M123 at Atmospheric Pressure?", "Is BeamDump at Atmospheric Pressure?", "Is OAP at Atmospheric Pressure?", "Is BLT at Atmospheric Pressure", "Is TARGET at Atmospheric Pressure?", "Is BLT2 at Atmospheric Pressure?", "Is HPD at Atmospheric Pressure?", "Is the EC Roughing Pump ON?", "Is the EC Roughing Pump OFF?", "Does the EC Roughing Pump have a fault?", "Is the LB Roughing Pump ON?", "Is the LB Roughing Pump Off?", "Does the LB Roughing Pump have a fault?", "Is the EC Backing Pump ON?", "Is the EC Backing Pump OFF?", "Is the LB Backing Pump ON?", "Is the LB Backing Pump OFF?", "Does the EC Backing Pump have a fault?", "Does the LB Backing Pump have a fault?", "Is the EC Backing Pipe at Atmospheric Pressure", "Is the LB Backing Pipe at Atmospheric Pressure", "Is the EC Backing Manifold at Atmospheric Pressure", "s the LB Backing Manifold at Atmospheric Pressure?", "Is the EC Roughing Pipe at Atmospheric Pressure", "Is the LB Roughing Pipe at Atmospheric Pressure?", "Is the EC Roughing Manifold at Atmospheric Pressure", "Is the LB Roughing Manifold at Atmospheric Pressure", "Is LB Backing Manifold Valve Opened?", "Is EC Backing Manifold Valve Opened?", "Is LB Roughing Manifold Valve Opened?", "Is EC Roughing Manifold Valve Opened?", "Is COMP Roughing Valve Opened?", "Is M123 Roughing Valve Opened?", "Is M123 Roughing Valve Closed?", "Is OAP Roughing Valve Opened?", "Is OAP Roughing Valve Closed?", "Is HPBD Roughing Valve Opened?", "Is HPBD Roughing Valve Closed?", "Is BTL Roughing Valve Opened?", "Is BTL Roughing Valve Closed?", "Is TARGET Roughing Valve Opened?", "Is TARGET Roughing Valve Closed?", "Is BTL2 Roughing Valve Opened?", "Is BTL2 Roughing Valve Closed?", "Is HPD Roughing Valve Opened?", "Is HPD Roughing Valve Closed?", "Is COMP Turbo Backing Valve Opened?", "Is M123 Turbo Backing Valve Opened", "Is HPBD Turbo Backing Valve Opened?", "Is OAP Turbo Backing Valve Opened?", "Is BTL Turbo Backing Valve Opened?", "Is TARGET1 Turbo Backing Valve Opened?", "Is TARGET2 Turbo Backing Valve Opened?", "Is BTL2 Turbo Backing Valve Opened?", "Is HPD Turbo Backing Valve Opened?", "Is M123 Backing at MID-VAC?", "Is OAP Backing at MID-VAC?", "Is TARGET1 Backing at MID-VAC?", "Is TARGET2 Backing at MID-VAC?", "Is BTL Backing at MID-VAC?", "Is BTL2 Backing at MID-VAC?", "Is HPD Backing at MID-VAC?", "Is M123 Turbo in Normal Operation", "Is COMP Turbo in Normal Operation", "Is OAP Turbo in Normal Operation", "Is BTL Turbo in Normal Operation", "Is TARGET1 Turbo in Normal Operation", "Is TARGET2 Turbo in Normal Operation", "Is BTL2 Turbo in Normal Operation", "Is HPD Turbo in Normal Operation", "Is M123 at MID-VAC?", "Is OAP at MID-VAC?", "Is COMP at MID-VAC?", "Is BTL at MID-VAC?", "Is TARGET at MID-VAC?", "Is BTL2 at MID-VAC?", "Is HPD at MID-VAC?"]
        w1912 = T32[] [enum."Is the EC Backing Pump ON?", enum."Does the EC Backing Pump have a fault?"] items=["No Action", "Is EC GPM Mode ON?", "Is EC GPM Mode Off?", "Is EC GVM Mode ON?", "Is EC GVM Off?", "Is  EC GPM or GVM Mode ON?", "Is LB GPM Mode ON?", "Is LB GPM Mode Off?", "Is LB GVM Mode ON?", "Is LB GVM Mode Off?", "Is  LB GPM or GVM Mode ON?", "Is M123 Turbo Gate Valve Opened? ", "Is M123 Turbo Gate Valve Closed?", "Is OAP Turbo Gate Valve Opened?", "Is OAP Turbo Gate Valve Closed?", "Is BTLTurbo Gate Valve Opened?", "Is BTL Turbo Gate Valve Closed?", "Is TARGET Turbo Gate Valve 1Opened?", "Is TARGET1 Turbo Gate Valve Closed?", "Is TARGET Turbo Gate Valve 2 Opened?", "Is TAREGT2 Turbo Gate Valve Closed?", "Is BTL2 Turbo Gate Valve Opened?", "Is BTL2 Turbo Gate Valve Closed?", "Is HPD Turbo Gate Valve Opened?", "Is HPD Turbo Gate Valve Closed?", "Is COMP to M123 gate Valve Opened?", "Is COMP to M123 Valve Closed?", "Is HPBD Gate Valve Opened?", "Is HPBD Gate Valve Closed?", "Is M123 to OAP gate valve opened?", "Is M123 to OAP gate valve closed?", "Is OAP to BLT gate valve opened?", "Is OAP to BTL Gate Valve Closed?", "Is BLT to TARGET gate valve opened?", "Is BTL to TARGET Gate Valve Closed?", "Is TARGET to BLT2 gate valve opened?", "Is TARGET to BTL2 Gate Valve Closed?", "Is BLT2 to HPD gate valve opened?", "Is BTL2 to HPD Gate Valve Closed?", "Is COMP at Atmospheric Pressure?", "Is M123 at Atmospheric Pressure?", "Is BeamDump at Atmospheric Pressure?", "Is OAP at Atmospheric Pressure?", "Is BLT at Atmospheric Pressure", "Is TARGET at Atmospheric Pressure?", "Is BLT2 at Atmospheric Pressure?", "Is HPD at Atmospheric Pressure?", "Is the EC Roughing Pump ON?", "Is the EC Roughing Pump OFF?", "Does the EC Roughing Pump have a fault?", "Is the LB Roughing Pump ON?", "Is the LB Roughing Pump Off?", "Does the LB Roughing Pump have a fault?", "Is the EC Backing Pump ON?", "Is the EC Backing Pump OFF?", "Is the LB Backing Pump ON?", "Is the LB Backing Pump OFF?", "Does the EC Backing Pump have a fault?", "Does the LB Backing Pump have a fault?", "Is the EC Backing Pipe at Atmospheric Pressure", "Is the LB Backing Pipe at Atmospheric Pressure", "Is the EC Backing Manifold at Atmospheric Pressure", "s the LB Backing Manifold at Atmospheric Pressure?", "Is the EC Roughing Pipe at Atmospheric Pressure", "Is the LB Roughing Pipe at Atmospheric Pressure?", "Is the EC Roughing Manifold at Atmospheric Pressure", "Is the LB Roughing Manifold at Atmospheric Pressure", "Is LB Backing Manifold Valve Opened?", "Is EC Backing Manifold Valve Opened?", "Is LB Roughing Manifold Valve Opened?", "Is EC Roughing Manifold Valve Opened?", "Is COMP Roughing Valve Opened?", "Is M123 Roughing Valve Opened?", "Is M123 Roughing Valve Closed?", "Is OAP Roughing Valve Opened?", "Is OAP Roughing Valve Closed?", "Is HPBD Roughing Valve Opened?", "Is HPBD Roughing Valve Closed?", "Is BTL Roughing Valve Opened?", "Is BTL Roughing Valve Closed?", "Is TARGET Roughing Valve Opened?", "Is TARGET Roughing Valve Closed?", "Is BTL2 Roughing Valve Opened?", "Is BTL2 Roughing Valve Closed?", "Is HPD Roughing Valve Opened?", "Is HPD Roughing Valve Closed?", "Is COMP Turbo Backing Valve Opened?", "Is M123 Turbo Backing Valve Opened", "Is HPBD Turbo Backing Valve Opened?", "Is OAP Turbo Backing Valve Opened?", "Is BTL Turbo Backing Valve Opened?", "Is TARGET1 Turbo Backing Valve Opened?", "Is TARGET2 Turbo Backing Valve Opened?", "Is BTL2 Turbo Backing Valve Opened?", "Is HPD Turbo Backing Valve Opened?", "Is M123 Backing at MID-VAC?", "Is OAP Backing at MID-VAC?", "Is TARGET1 Backing at MID-VAC?", "Is TARGET2 Backing at MID-VAC?", "Is BTL Backing at MID-VAC?", "Is BTL2 Backing at MID-VAC?", "Is HPD Backing at MID-VAC?", "Is M123 Turbo in Normal Operation", "Is COMP Turbo in Normal Operation", "Is OAP Turbo in Normal Operation", "Is BTL Turbo in Normal Operation", "Is TARGET1 Turbo in Normal Operation", "Is TARGET2 Turbo in Normal Operation", "Is BTL2 Turbo in Normal Operation", "Is HPD Turbo in Normal Operation", "Is M123 at MID-VAC?", "Is OAP at MID-VAC?", "Is COMP at MID-VAC?", "Is BTL at MID-VAC?", "Is TARGET at MID-VAC?", "Is BTL2 at MID-VAC?", "Is HPD at MID-VAC?"]
        w1922 = "Main: Wait for Backing Pump"
        w1928 = Error_codes."007-Backing Pump Status" ("Error Codes")
        # "Event TAG"
        n750 = Unbundle By Name(w1914) -> ("Chamber Selection"=w1913:T21)
        n751 = call "Selection ActionBuilder sections.vi"("EC Query Array"=w1912, "LB Query Array"=w1911, "Chamber Selection"=w1913) -> ("Query Array out"=w1910:T32[])  [unwired: 7 in, 1 out]
        n752 = call "GetAction.vi"("Check Condition"=w1928, "Query Array"=w1910) -> ("Status Array Out"=w1929:string[], "Generate Event?"=w1920:bool, "error out"=w1927:errorcluster)  [unwired: 8 in, 3 out]
        n753 = call "Generate User Event.vi"("Add(t)/Remove(f) Event"=w1920, "error in (no error)"=w1927, "User Event in"=w1918, "Status Array In"=w1929, "Error Codes"=w1928) -> ()  [unwired: 5 in, 2 out]
        n754 = call "MID-VAC Timer.vi"("Action"=timerAction_typdef."Timer Running") -> ("TO"=w1925:bool)  [unwired: 10 in]
        n755 = And(x=w1920, y=w1925) -> (x .and. y?=w1924:bool)
        n756 = Unbundle By Name(w1914) -> ()  [unwired: 1 out]
        n757 = control-ref of="User Input Panel"() -> (w1923:refnum<vi>)
        n758 = call "Generate TO event.vi"("Boolean"=w1924, "message"="Backing Pump is NOT On or has a fault.\nClick Continue to Wait for 30 Seconds.\nClick Exit to abort GPM", "User Event in"=w1917) -> ()  [unwired: 9 in]
        n759 = call "Gen Next State based on user input.vi"("Next State IN"="Main: Wait for MID-VAC on backing pressure", "Generate Event?"=w1920, "Idle State"=w1922, "Timer before next step (20s)"=600.0, "Continue To Wait State"=w1922, "SubPanel in"=w1923) -> ("Next State Out"=w1916:string)  [unwired: 5 in]
        n760 = call <vilib>:"Add State(s) to Queue__jki_lib_state_machine.vi"("State(s) in Front (\"\")"=w1916, "State(s) in (\"\")"=w1931) -> ("States Out"=w1932:string)  [unwired: 13 in]
      }
      frame "Main: Wait for MID-VAC on backing pressure" {
        w1945 = "Main: Wait for MID-VAC on backing pressure"
        w1952 = Error_codes."013-MID-VAC Status" ("Error Codes")
        # "Event TAG"
        n761 = Unbundle By Name(w1934) -> ("Chamber Selection"=w1937:T21, "Isolate HPBD"=w1935:bool)
        n762 = call "Selection ActionBuilder.vi"("Selection Action"=Selection_Action_typdef."Check MID-VAC on Chambers", "Isolate HPBD"=w1935, "Chamber Selection"=w1937) -> ("Action Array Out"=w1933:T32[])  [unwired: 7 in, 1 out]
        n763 = call "GetAction.vi"("Check Condition"=w1952, "Query Array"=w1933, "input cluster"=w1934, "error in (no error)"=w1954) -> ("Status Array Out"=w1953:string[], "Generate Event?"=w1940:bool, "error out"=w1950:errorcluster)  [unwired: 6 in, 3 out]
        n764 = call "MID-VAC Timer.vi"("Action"=timerAction_typdef."Timer Running") -> ("TO"=w1947:bool)  [unwired: 10 in]
        n765 = call "Generate User Event.vi"("Add(t)/Remove(f) Event"=w1940, "error in (no error)"=w1950, "User Event in"=w1951, "Status Array In"=w1953, "Error Codes"=w1952) -> ("error out"=w1949:errorcluster)  [unwired: 5 in, 1 out]
        n766 = And(x=w1940, y=w1947) -> (x .and. y?=w1941:bool)
